vi "FindSupportedModules.vi"(11 "Device Model":T1) -> (0 "Last Dynamic Module":string, 1 "Channels per Supported Module":i32[](array[numeric])=[3, 3, 3, 4, 4], 2 "All Supported Modules":string[](array[string]), 3 "Number of Supported Modules":i32)   [LabVIEW 2017, in "CmsAcquisition.lvlib"]
uses:
  <vilib>/addons/InsightCM/Devices/Shared/Cms/CmsAcquisition/CmsAcquisition.lvlib
  <vilib>/addons/InsightCM/MessageBus/Base/controls/R2_Device.ctl
  <vilib>/addons/InsightCM/MessageBus/Base/controls/KeyValuePair.ctl
  <vilib>/addons/InsightCM/MessageBus/Base/controls/DeviceState.ctl
  <vilib>/addons/InsightCM/MessageBus/Base/controls/R2_DataGroup.ctl
  <vilib>/addons/InsightCM/MessageBus/Base/controls/OperatingState.ctl
  <vilib>/addons/InsightCM/MessageBus/Base/controls/Trigger.ctl
  <vilib>/addons/InsightCM/MessageBus/Base/controls/Condition.ctl
  <vilib>/addons/InsightCM/MessageBus/Base/controls/BurstModeTrigger.ctl
  <vilib>/addons/InsightCM/MessageBus/Base/controls/DeviceSensorGroup.ctl
  <vilib>/addons/InsightCM/MessageBus/Base/controls/WirelessEndpoint.ctl
  <vilib>/addons/InsightCM/MessageBus/Base/controls/WirelessChannel.ctl
  <vilib>/addons/InsightCM/Utilities/DeviceModelHelpers/DeviceModelHelpers.lvlib
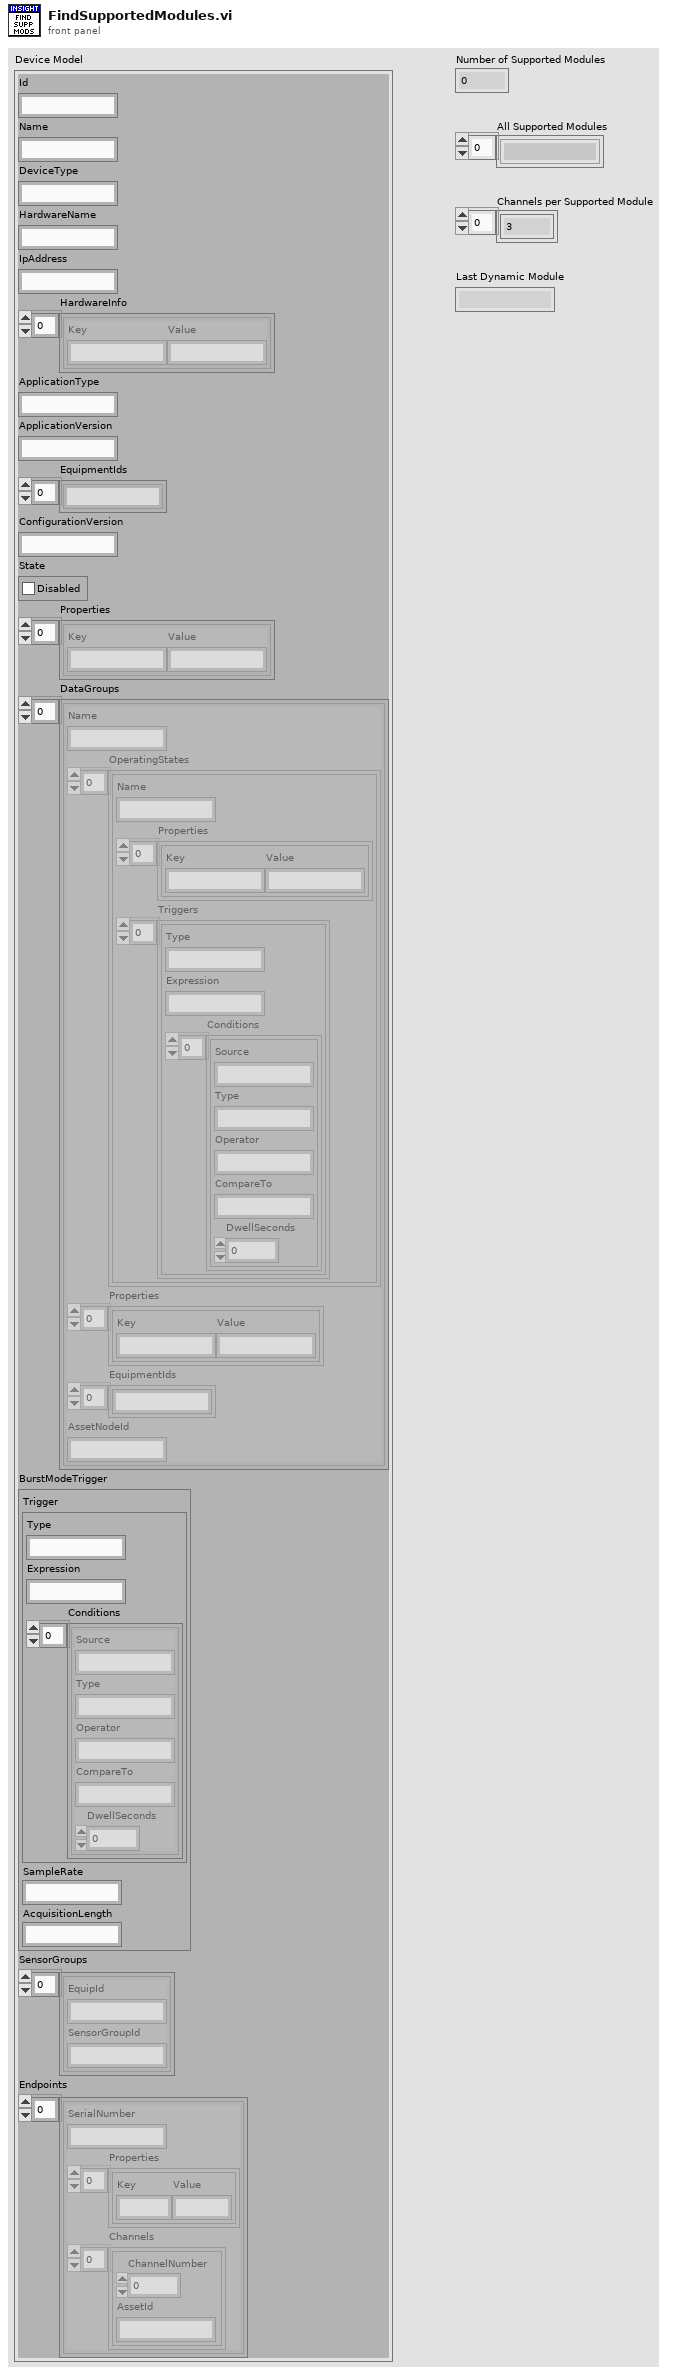
[diagram p1: front panel]
types:
  T1 = typedef "R2_Device.ctl" = cluster{"Id":string, "Name":string, "DeviceType":string, "HardwareName":string, "IpAddress":string, "HardwareInfo":T2[], "ApplicationType":string, "ApplicationVersion":string, "EquipmentIds":string[], "ConfigurationVersion":string, "State":T3, "Properties":T2[], "DataGroups":T4[], "BurstModeTrigger":T8, "SensorGroups":T9[], "Endpoints":T10[]}
  T2 = typedef "KeyValuePair.ctl" = cluster{"Key":string, "Value":string}
  T3 = typedef "DeviceState.ctl" = cluster{"Disabled":bool}
  T4 = typedef "R2_DataGroup.ctl" = cluster{"Name":string, "OperatingStates":T5[], "Properties":T2[], "EquipmentIds":string[], "AssetNodeId":string}
  T5 = typedef "OperatingState.ctl" = cluster{"Name":string, "Properties":T2[], "Triggers":T6[]}
  T6 = typedef "Trigger.ctl" = cluster{"Type":string, "Expression":string, "Conditions":T7[]}
  T7 = typedef "Condition.ctl" = cluster{"Source":string, "Type":string, "Operator":string, "CompareTo":string, "DwellSeconds":dbl}
  T8 = typedef "BurstModeTrigger.ctl" = cluster{"Trigger":T6, "SampleRate":string, "AcquisitionLength":string}
  T9 = typedef "DeviceSensorGroup.ctl" = cluster{"EquipId":string, "SensorGroupId":string}
  T10 = typedef "WirelessEndpoint.ctl" = cluster{"SerialNumber":string, "Properties":T2[], "Channels":T11[]}
  T11 = typedef "WirelessChannel.ctl" = cluster{"ChannelNumber":i32, "AssetId":string}
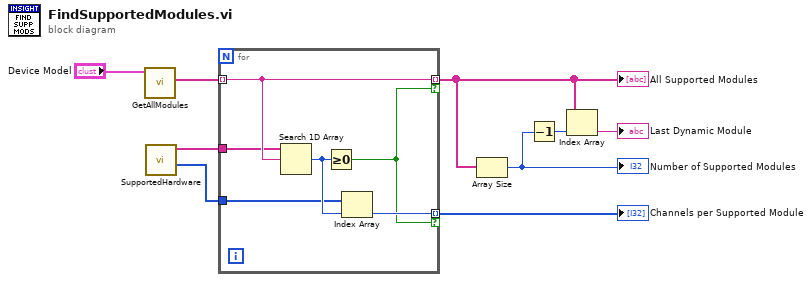
[diagram p0: block diagram]
diagram:
  n1 = call <vilib>:"GetAllModules.vi"("device in"="Device Model") -> ("all modules"=w8:string[])  [unwired: 9 in, 1 out]
  n2 = call <vilib>:"SupportedHardware.vi"() -> ("Channels per Module"=w6:i32[], "Supported Hardware"=w7:string[])  [unwired: 10 in]
  n3 = for {
    tunnel: w8 -> [w15] mode=indexing
    tunnel: [w15] -> w1 mode=indexing if=w10
    tunnel: w7 -> [w14]
    tunnel: w6 -> [w12]
    tunnel: [w11] -> w5 mode=indexing if=w10
    n4 = Search 1D Array(1D array=w14, element=w15) -> (index of element=w13:i32)  [unwired: 1 in]
    n5 = Greater Or Equal To 0?(x=w13) -> (x >= 0?=w10:bool)
    n6 = Index Array(array=w12, index=w13) -> (element=w11:i32)
  }
  "All Supported Modules" <- w1
  "Channels per Supported Module" <- w5
  n7 = Array Size(array=w1) -> (size(s)=w4:i32)
  "Number of Supported Modules" <- w4
  n8 = Decrement(x=w4) -> (x-1=w3:i32)
  n9 = Index Array(array=w1, index=w3) -> (element=→"Last Dynamic Module":string)
